vi "Performance Test.vi"() -> ()   [LabVIEW 2021]
uses:
  <vilib>/Platform/TimedLoop/XDataNode/wakeup.ctl
  <vilib>/Platform/TimedLoop/XDataNode/XDNodeRunTimeDep.lvlib
  <vilib>/Platform/TimedLoop/XDataNode/nitl_modes.ctl
  <vilib>/Platform/TimedLoop/XDataNode/timing_clust.ctl
  <vilib>/Platform/TimedLoop/XDataNode/XDataNode.xnode
  CIFChannels/Typedef/Direction.ctl
  CIFChannels/CIFChannels.lvclass
  ChannelCommon/typedef/FIFO Config.ctl
  ChannelCommon/ChannelCommon.lvlib
  ChannelRegistrar/typedef/Datatype CAN.ctl
  ChannelRegistrar/ChannelRegistrar.lvlib
  CIF_NIChn_FifoCAN.lvclass
  D:/dev/CIF-LVCore/src/Channels/CIF_NIChn/NIChn/CIF_NIChn.lvclass
  D:/dev/CIF-LVCore/src/Channels/CIFChannels/CIFChannels.lvclass
  D:/dev/CIF-LVCore/src/Channels/CIF_NIChn/FIFO_CAN/CIF_NIChn_FifoCAN.lvclass
panel:
  out "avg CAN_TO":dbl
  out "max CAN_TO":dbl
  out "timed out? 3":bool
  out "avg CAN_Direct":dbl
  out "max CAN_Direct":dbl
  out "timed out? 2":bool
  out "timed out?":bool
  out "avg CAN channel":dbl
  out "max CAN channel":dbl
  out "pass":bool
  out "error out":errorcluster
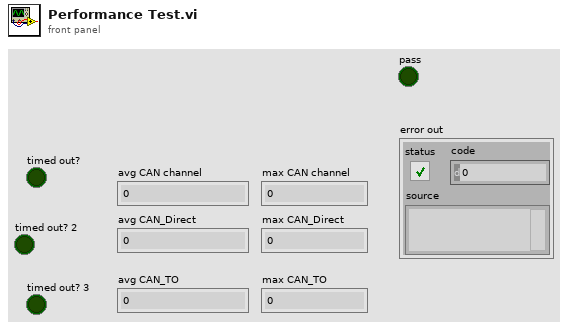
[diagram p1: front panel]
types:
  T1 = typedef "ChannelCommon.lvlib/FIFO Config.ctl" = cluster{"Depth":u64, "Flags":u64}
  T2 = typedef "CIFChannels.lvclass/Direction.ctl" = enum16{"Publisher", "Subscriber"}
  T3 = typedef "ChannelRegistrar.lvlib/Datatype CAN.ctl" = cluster{"payload":u8[], "identifier":u32, "Tags":u8, "Timestamp":u64}
  T4 = typedef "XDNodeRunTimeDep.lvlib/timing_clust.ctl" = cluster{"Expected End [f-1]":u64, "Actual End [f-1]":u64, "Finished Late? [f-1]":bool, "Expected End [i-1]":u64, "Actual End [i-1]":u64, "Finished Late? [i-1]":bool, "Expected Start [i]":u64, "Actual Start [i]":u64, "Expected Start [f]":u64, "Actual Start [f]":u64, "Source Name":string, "Structure Name":string, "Period":i64, "Deadline":i64, "Offset":i64, "Start":i64, "Priority":i32, "Timeout":i32, "Mode":T5, "Wakeup Reason":T6, "Error":errorcluster, "Source Type":string, "Secondary Source Type":string, "Global End Time":u64, "Global Start Time":u64, "Frame Duration":u64, "Iteration Duration":u64, "Assigned CPU":i32, "I/O Scan Engine Mode":u32}
  T5 = typedef "XDNodeRunTimeDep.lvlib/nitl_modes.ctl" = enum32{"No Change", "Process missed periods, maintain original phase", "Discard missed periods, maintain original phase", "Process missed periods, ignore original phase", "Discard missed periods, ignore original phase"}
  T6 = typedef "XDNodeRunTimeDep.lvlib/wakeup.ctl" = enum32{"Normal", "Aborted", "Asynchronous wakeup", "Timing source error", "Timed loop error", "Timeout"}
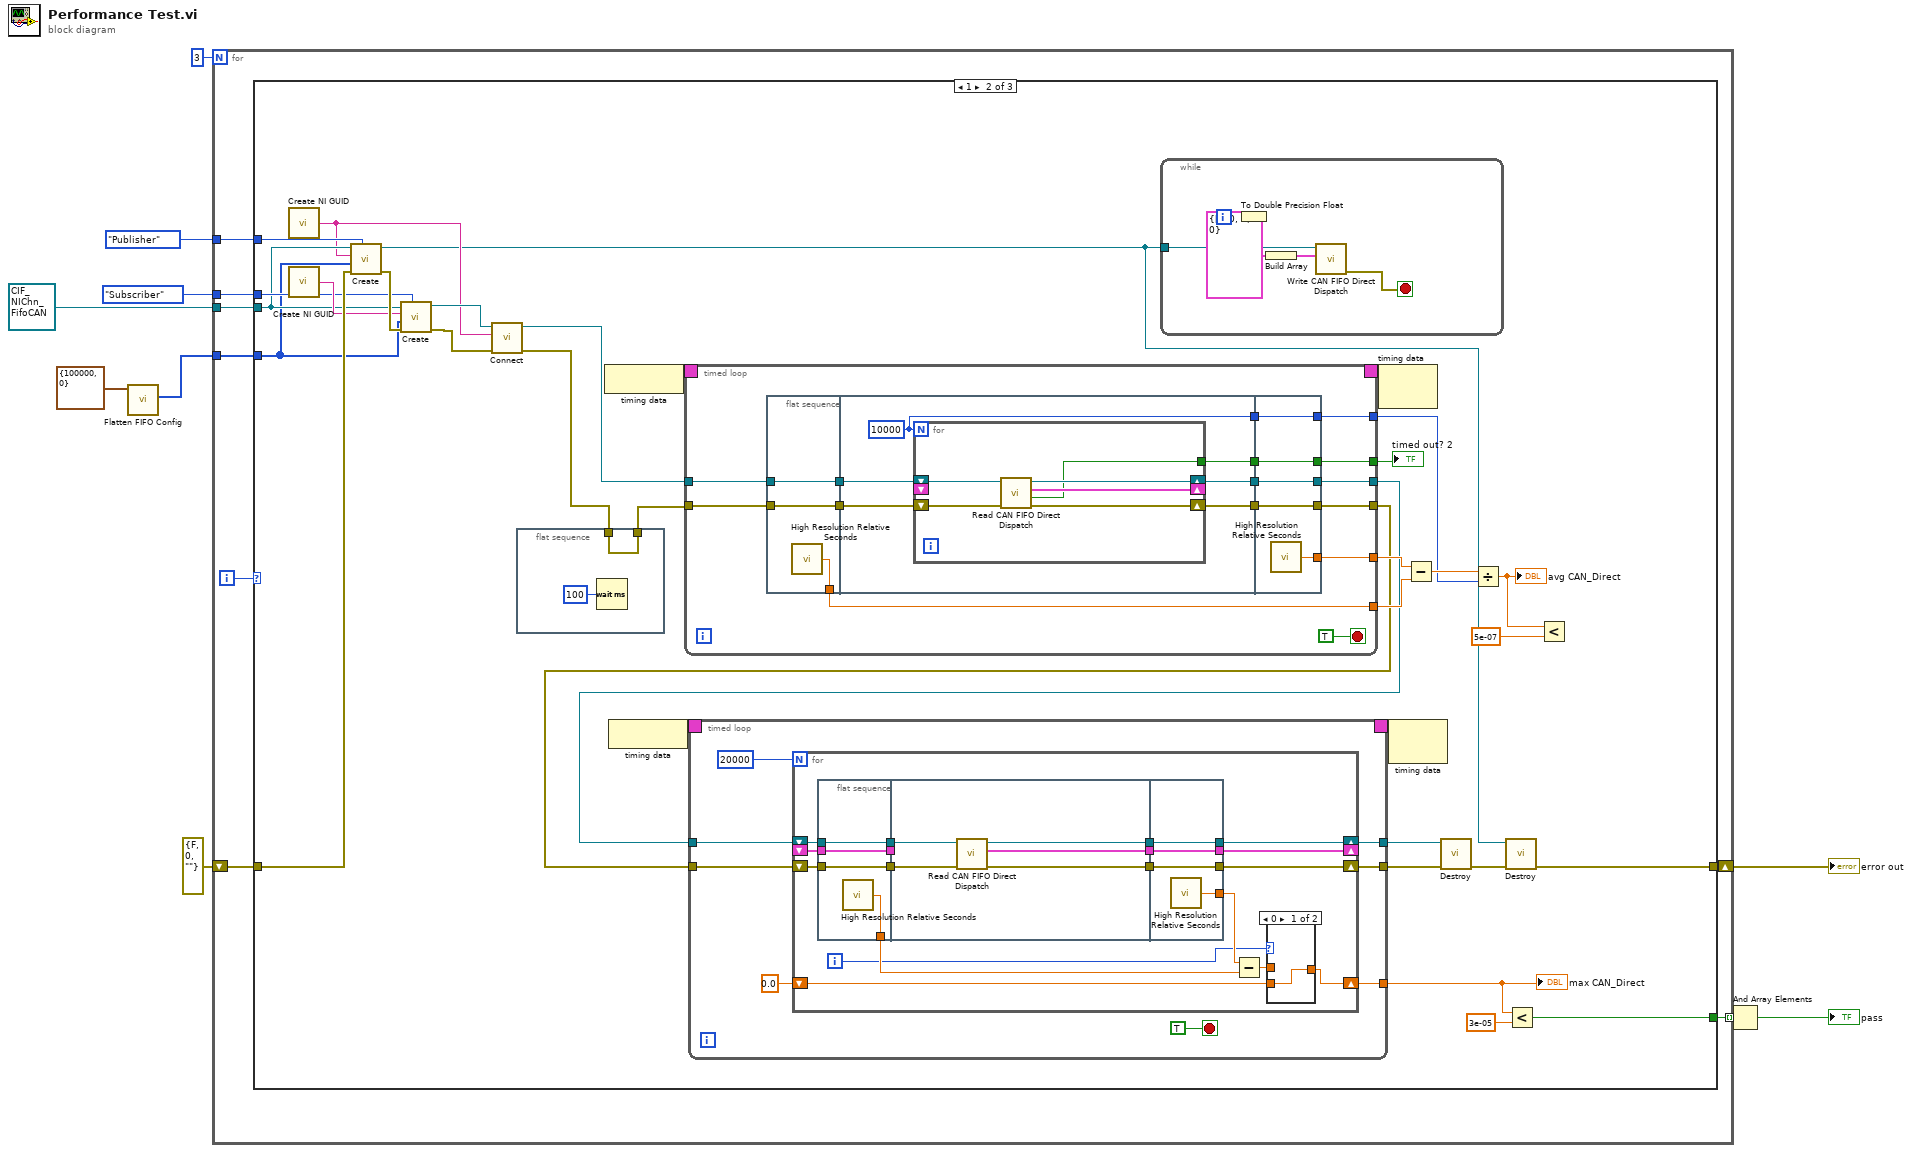
[diagram p0: block diagram]
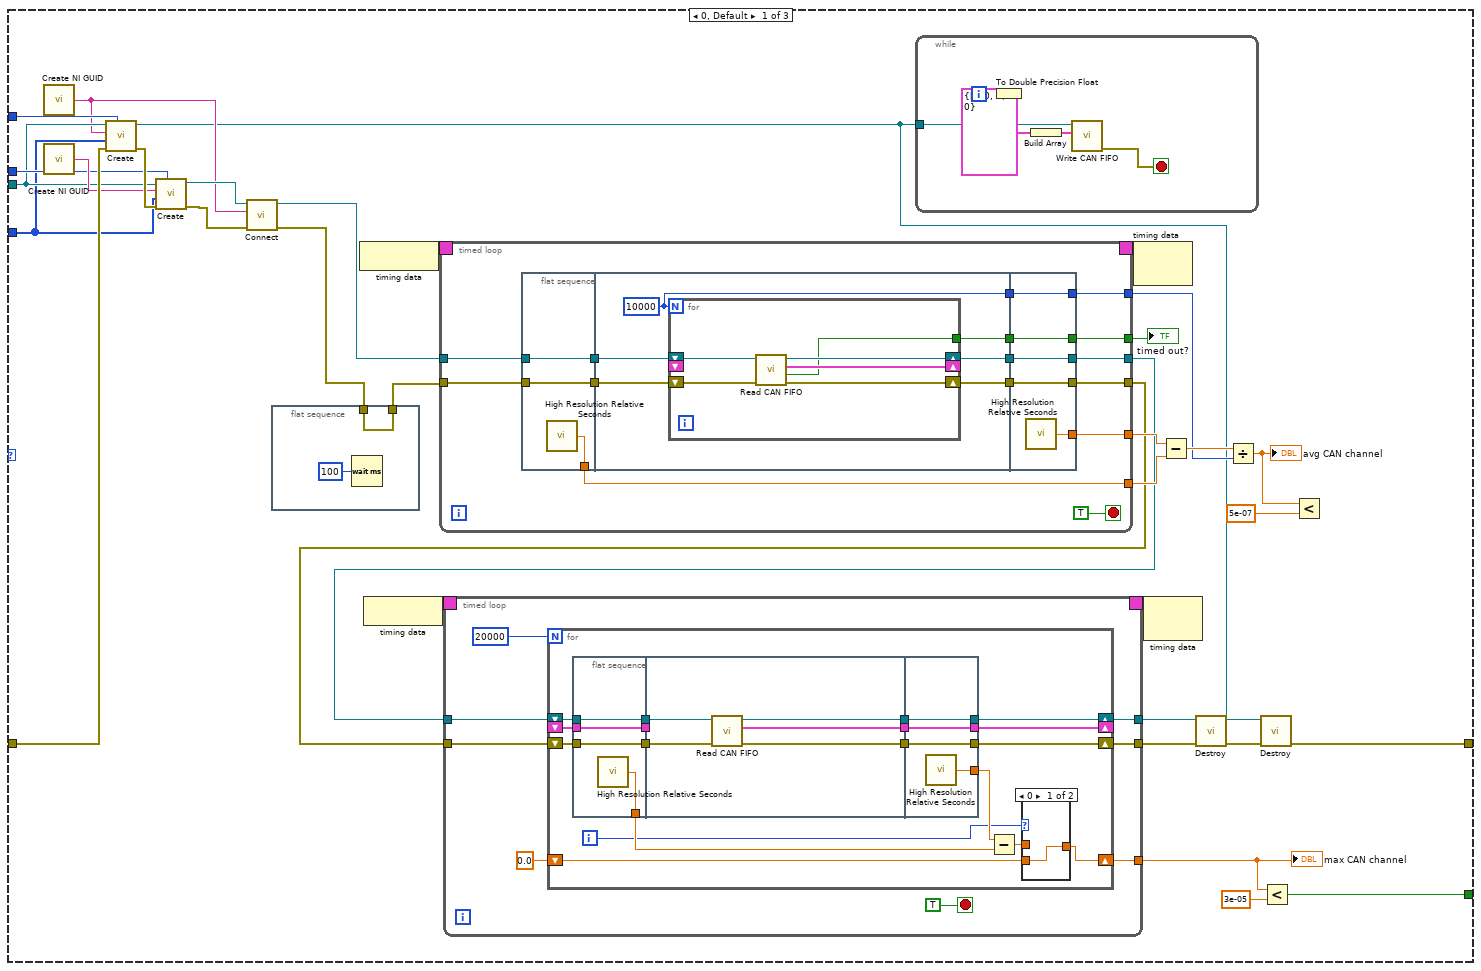
[diagram p2: hidden frame]
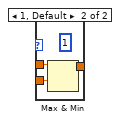
[diagram p3: hidden frame]
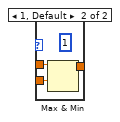
[diagram p4: hidden frame]
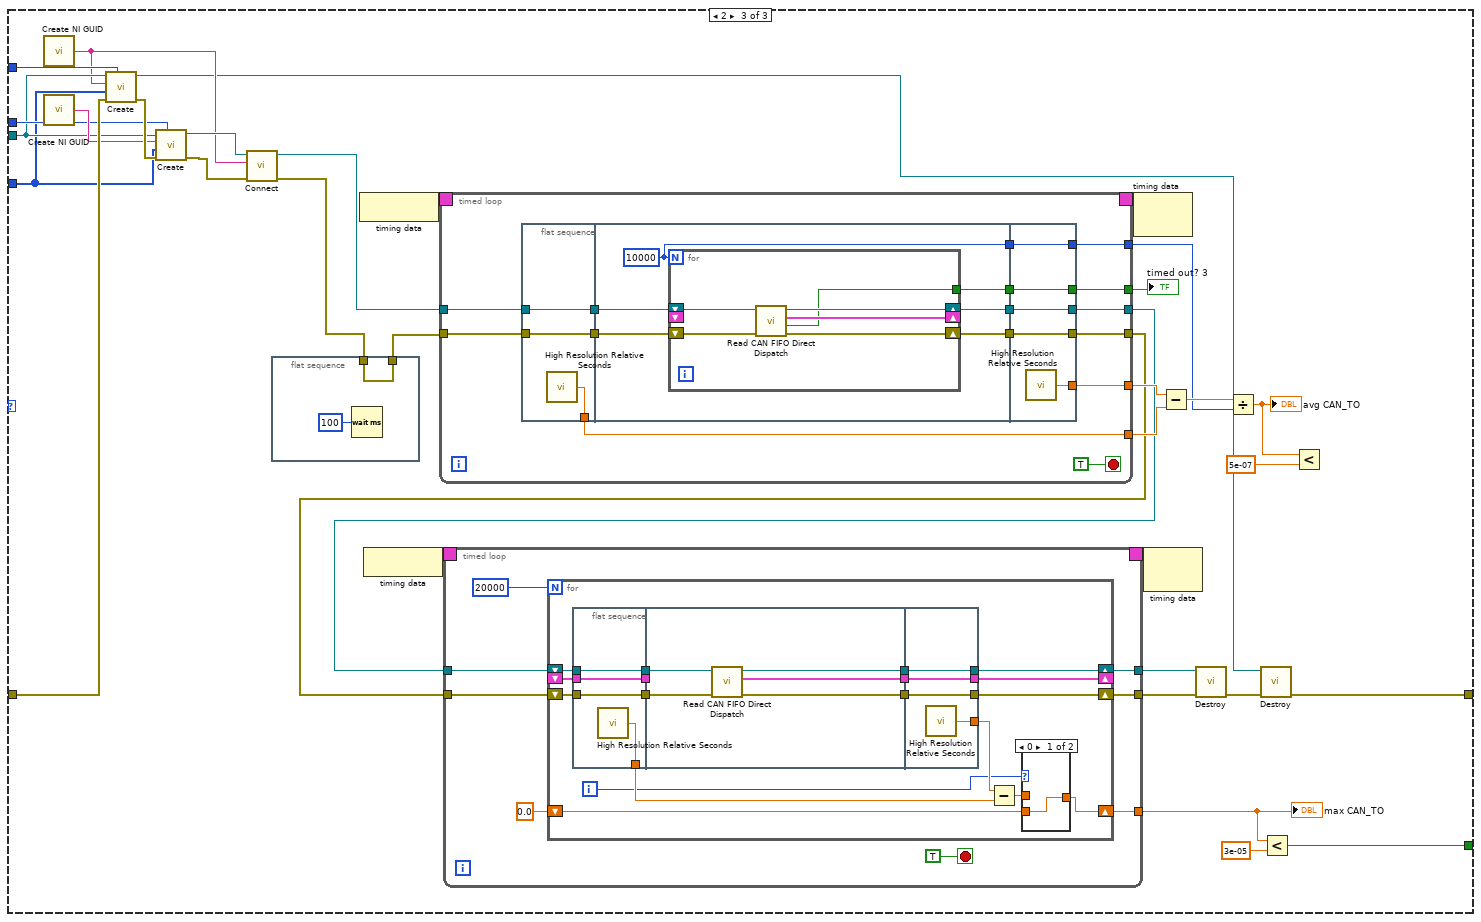
[diagram p5: hidden frame]
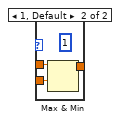
[diagram p6: hidden frame]
diagram:
  n1 = call "Flatten FIFO Config.vi"("FIFO Config in"=T1 {"Depth"=100000, "Flags"=0}) -> ("Flattened Data out"=w2:u8[])  [unwired: 8 in, 2 out]
  n2 = for {
    N: 3 -> [_]
    tunnel: [w18] -> w8 mode=indexing
    shift-right: [w17] -> w10
    shift-left: errorcluster {"status"=FALSE, "code"=0, "source"=""} ("error out") -> [w15]
    tunnel: Direction."Publisher" ("Direction") -> [w14]
    tunnel: Direction."Subscriber" ("Direction") -> [w13]
    tunnel: refnum<class "CIF_NIChn_FifoCAN.lvclass"> refnum ("CIF_NIChn_FifoCAN.lvclass") -> [w12]
    tunnel: w2 -> [w11]
    i -> [w16]
    n3 = case shown="1" w16 {
      tunnel: [w38 w165 w292] -> w18
      tunnel: [w22 w149 w276] -> w17
      tunnel: w15 -> [w36 w163 w290]
      tunnel: w14 -> [w34 w161 w288]
      tunnel: w13 -> [w33 w160 w287]
      tunnel: w12 -> [w32 w159 w286]
      tunnel: w11 -> [w28 w155 w282]
      frame 0, Default {
        n4 = call <vilib>:"Create NI GUID.vi"() -> ("NI GUID"=w30:string)
        n5 = call <vilib>:"Create NI GUID.vi"() -> ("NI GUID"=w35:string)
        n6 = call-dynamic "Create.vi"("Direction"=w34, "error in (no error)"=w36, "Custom Config Data"=w28, "Name"=w30, "CIFTag in"=w32) -> ("error out"=w37:errorcluster, "CIFTag out"=w23:refnum<class "CIF_NIChn_FifoCAN.lvclass">)  [unwired: 5 in]
        n7 = call-dynamic "Create.vi"("Direction"=w33, "error in (no error)"=w37, "Custom Config Data"=w28, "Name"=w35, "CIFTag in"=w32) -> ("error out"=w29:errorcluster, "CIFTag out"=w31:refnum<class "CIF_NIChn_FifoCAN.lvclass">)  [unwired: 5 in]
        n8 = call-dynamic "Connect.vi"("error in (no error)"=w29, "Connection Name"=w30, "CIFTag in"=w31) -> ("error out"=w21:errorcluster, "CIFTag out"=w27:refnum<class "CIF_NIChn_FifoCAN.lvclass">)  [unwired: 7 in]
        n9 = flat-sequence {
          tunnel: w21 -> [w54]
          tunnel: [w54] -> w20
          frame #0 {
            n10 = Wait (ms)(milliseconds to wait=u32 100) -> ()  [unwired: 1 out]
          }
        }
        n11 = node-c288() -> (w52:T4)
        n12 = node-c288() -> (w50:T4)
        n13 = timed-loop {
          timing: w52 -> [_]
          timing-out: [_] -> w51
          tunnel: w27 -> [w121]
          tunnel: w20 -> [w120]
          tunnel: [w116] -> w44
          tunnel: [w114] -> w43
          tunnel: [w112] -> w48
          tunnel: [w111] -> w47
          tunnel: [w110] -> w45
          tunnel: [w108] -> w19
          stop <- TRUE stop-if-true
          n14 = flat-sequence {
            tunnel: w120 -> [w123]
            tunnel: w121 -> [w124]
            tunnel: [w124] -> w118
            tunnel: [w123] -> w117
            tunnel: [w122] -> w111
            tunnel: w118 -> [w130]
            tunnel: w117 -> [w129]
            tunnel: [w128] -> w115
            tunnel: [w127] -> w113
            tunnel: [w126] -> w109
            tunnel: [w125] -> w107
            tunnel: [w141] -> w116
            tunnel: w115 -> [w141]
            tunnel: [w140] -> w114
            tunnel: w113 -> [w140]
            tunnel: [w139] -> w112
            tunnel: [w138] -> w110
            tunnel: w109 -> [w138]
            tunnel: [w137] -> w108
            tunnel: w107 -> [w137]
            frame #0 {
              n15 = call <vilib>:"High Resolution Relative Seconds.vi"() -> ("relative seconds"=w122:dbl)
            }
            frame #1 {
              w126 = 10000
              n16 = for {
                N: w126 -> [_]
                shift-right: [w135] -> w128
                shift-left: w130 -> [w136]
                shift-right: [w133] -> w127
                shift-left: w129 -> [w134]
                shift-right: [w132] -> _
                shift-left: _ -> [_]
                tunnel: [w131] -> w125
                n17 = call-dynamic "Read CAN FIFO.vi"("error in (no error)"=w134, "CIFTag in"=w136) -> ("error out"=w133:errorcluster, "timed out?"=w131:bool, "Data"=w132:T3[], "CIFTag out"=w135:refnum<class "CIF_NIChn_FifoCAN.lvclass">)  [unwired: 5 in, 1 out]
              }
            }
            frame #2 {
              n18 = call <vilib>:"High Resolution Relative Seconds.vi"() -> ("relative seconds"=w139:dbl)
            }
          }
        }
        "timed out?" <- w19
        n19 = timed-loop {
          timing: w50 -> [_]
          timing-out: [_] -> w49
          tunnel: w44 -> [w67]
          tunnel: w43 -> [w66]
          tunnel: [w64] -> w26
          tunnel: [w63] -> w25
          tunnel: [w60] -> w40
          stop <- TRUE stop-if-true
          n20 = for {
            N: 20000 -> [_]
            shift-right: [w79] -> w64
            shift-left: w67 -> [w81]
            shift-right: [w78] -> w63
            shift-left: w66 -> [w80]
            shift-right: [w72] -> w60
            shift-left: 0.0 -> [w73]
            shift-right: [w71] -> _
            shift-left: _ -> [w77]
            i -> [w69]
            n21 = flat-sequence {
              tunnel: w80 -> [w92]
              tunnel: w81 -> [w93]
              tunnel: [w93] -> w85
              tunnel: [w92] -> w84
              tunnel: [w91] -> w75
              tunnel: w77 -> [w90]
              tunnel: [w90] -> w83
              tunnel: w85 -> [w98]
              tunnel: w84 -> [w96]
              tunnel: [w97] -> w82
              tunnel: w83 -> [_]
              tunnel: [w94] -> w70
              tunnel: [w95] -> w68
              tunnel: [w102] -> w79
              tunnel: w82 -> [w102]
              tunnel: [w101] -> w78
              tunnel: [w100] -> w76
              tunnel: [w99] -> w71
              tunnel: w70 -> [w99]
              tunnel: w68 -> [w101]
              frame #0 {
                n22 = call <vilib>:"High Resolution Relative Seconds.vi"() -> ("relative seconds"=w91:dbl)
              }
              frame #1 {
                n23 = call-dynamic "Read CAN FIFO.vi"("error in (no error)"=w96, "CIFTag in"=w98) -> ("error out"=w95:errorcluster, "Data"=w94:T3[], "CIFTag out"=w97:refnum<class "CIF_NIChn_FifoCAN.lvclass">)  [unwired: 5 in, 2 out]
              }
              frame #2 {
                n24 = call <vilib>:"High Resolution Relative Seconds.vi"() -> ("relative seconds"=w100:dbl)
              }
            }
            n25 = Subtract(x=w76, y=w75) -> (x-y=w74:dbl)
            n26 = case shown="0" w69 {
              tunnel: w74 -> [_ w89]
              tunnel: w73 -> [w86 w88]
              tunnel: [w86 w87] -> w72
              frame 0 {
              }
              frame 1, Default {
                (unwired) u32 1 ("milliseconds to wait")
                n27 = Max & Min(x=w89, y=w88) -> (max(x,y)=w87:dbl)  [unwired: 1 out]
              }
            }
          }
        }
        "max CAN channel" <- w40
        n28 = while {
          tunnel: w23 -> [w58]
          i -> [w59]
          stop <- w56 stop-if-true
          n29 = To Double Precision Float(number=w59) -> ()  [unwired: 1 out]
          n30 = Build Array(T3 {"payload"=[], "identifier"=0, "Tags"=0, "Timestamp"=0} ("Data")) -> (w55:T3[])
          n31 = call-dynamic "Write CAN FIFO.vi"("Data"=w55, "CIFTag in"=w58) -> ("error out"=w56:errorcluster)  [unwired: 7 in, 2 out]
        }
        n32 = node-c288(w51) -> ()  [unwired: 1 out]
        n33 = node-c288(w49) -> ()  [unwired: 1 out]
        n34 = Subtract(x=w48, y=w47) -> (x-y=w46:dbl)
        n35 = call-dynamic "Destroy.vi"("error in (no error)"=w25, "CIFTag in"=w26) -> ("error out"=w24:errorcluster)  [unwired: 8 in, 1 out]
        n36 = Divide(x=w46, y=w45) -> (x/y=w42:dbl)
        "avg CAN channel" <- w42
        n37 = call-dynamic "Destroy.vi"("error in (no error)"=w24, "CIFTag in"=w23) -> ("error out"=w22:errorcluster)  [unwired: 8 in, 1 out]
        n38 = Less?(x=w40, y=3e-05) -> (x < y?=w38:bool)
        n39 = Less?(x=w42, y=5e-07) -> ()  [unwired: 1 out]
      }
      frame 1 {
        n40 = call <vilib>:"Create NI GUID.vi"() -> ("NI GUID"=w157:string)
        n41 = call <vilib>:"Create NI GUID.vi"() -> ("NI GUID"=w162:string)
        n42 = call-dynamic "Create.vi"("Direction"=w161, "error in (no error)"=w163, "Custom Config Data"=w155, "Name"=w157, "CIFTag in"=w159) -> ("error out"=w164:errorcluster, "CIFTag out"=w150:refnum<class "CIF_NIChn_FifoCAN.lvclass">)  [unwired: 5 in]
        n43 = call-dynamic "Create.vi"("Direction"=w160, "error in (no error)"=w164, "Custom Config Data"=w155, "Name"=w162, "CIFTag in"=w159) -> ("error out"=w156:errorcluster, "CIFTag out"=w158:refnum<class "CIF_NIChn_FifoCAN.lvclass">)  [unwired: 5 in]
        n44 = call-dynamic "Connect.vi"("error in (no error)"=w156, "Connection Name"=w157, "CIFTag in"=w158) -> ("error out"=w148:errorcluster, "CIFTag out"=w154:refnum<class "CIF_NIChn_FifoCAN.lvclass">)  [unwired: 7 in]
        n45 = flat-sequence {
          tunnel: w148 -> [w181]
          tunnel: [w181] -> w147
          frame #0 {
            n46 = Wait (ms)(milliseconds to wait=u32 100) -> ()  [unwired: 1 out]
          }
        }
        n47 = node-c288() -> (w179:T4)
        n48 = node-c288() -> (w177:T4)
        n49 = timed-loop {
          timing: w179 -> [_]
          timing-out: [_] -> w178
          tunnel: w154 -> [w248]
          tunnel: w147 -> [w247]
          tunnel: [w243] -> w171
          tunnel: [w241] -> w170
          tunnel: [w239] -> w175
          tunnel: [w238] -> w174
          tunnel: [w237] -> w172
          tunnel: [w235] -> w146
          stop <- TRUE stop-if-true
          n50 = flat-sequence {
            tunnel: w247 -> [w250]
            tunnel: w248 -> [w251]
            tunnel: [w251] -> w245
            tunnel: [w250] -> w244
            tunnel: [w249] -> w238
            tunnel: w245 -> [w257]
            tunnel: w244 -> [w256]
            tunnel: [w255] -> w242
            tunnel: [w254] -> w240
            tunnel: [w253] -> w236
            tunnel: [w252] -> w234
            tunnel: [w268] -> w243
            tunnel: w242 -> [w268]
            tunnel: [w267] -> w241
            tunnel: w240 -> [w267]
            tunnel: [w266] -> w239
            tunnel: [w265] -> w237
            tunnel: w236 -> [w265]
            tunnel: [w264] -> w235
            tunnel: w234 -> [w264]
            frame #0 {
              n51 = call <vilib>:"High Resolution Relative Seconds.vi"() -> ("relative seconds"=w249:dbl)
            }
            frame #1 {
              w253 = 10000
              n52 = for {
                N: w253 -> [_]
                shift-right: [w262] -> w255
                shift-left: w257 -> [w263]
                shift-right: [w260] -> w254
                shift-left: w256 -> [w261]
                shift-right: [w259] -> _
                shift-left: _ -> [_]
                tunnel: [w258] -> w252
                n53 = call "Read CAN FIFO Direct Dispatch.vi"("error in (no error)"=w261, "CIFTag in"=w263) -> ("error out"=w260:errorcluster, "timed out?"=w258:bool, "Data"=w259:T3[], "CIFTag out"=w262:refnum<class "CIF_NIChn_FifoCAN.lvclass">)  [unwired: 5 in, 1 out]
              }
            }
            frame #2 {
              n54 = call <vilib>:"High Resolution Relative Seconds.vi"() -> ("relative seconds"=w266:dbl)
            }
          }
        }
        "timed out? 2" <- w146
        n55 = timed-loop {
          timing: w177 -> [_]
          timing-out: [_] -> w176
          tunnel: w171 -> [w194]
          tunnel: w170 -> [w193]
          tunnel: [w191] -> w153
          tunnel: [w190] -> w152
          tunnel: [w187] -> w167
          stop <- TRUE stop-if-true
          n56 = for {
            N: 20000 -> [_]
            shift-right: [w206] -> w191
            shift-left: w194 -> [w208]
            shift-right: [w205] -> w190
            shift-left: w193 -> [w207]
            shift-right: [w199] -> w187
            shift-left: 0.0 -> [w200]
            shift-right: [w198] -> _
            shift-left: _ -> [w204]
            i -> [w196]
            n57 = flat-sequence {
              tunnel: w207 -> [w219]
              tunnel: w208 -> [w220]
              tunnel: [w220] -> w212
              tunnel: [w219] -> w211
              tunnel: [w218] -> w202
              tunnel: w204 -> [w217]
              tunnel: [w217] -> w210
              tunnel: w212 -> [w225]
              tunnel: w211 -> [w223]
              tunnel: [w224] -> w209
              tunnel: w210 -> [_]
              tunnel: [w221] -> w197
              tunnel: [w222] -> w195
              tunnel: [w229] -> w206
              tunnel: w209 -> [w229]
              tunnel: [w228] -> w205
              tunnel: [w227] -> w203
              tunnel: [w226] -> w198
              tunnel: w197 -> [w226]
              tunnel: w195 -> [w228]
              frame #0 {
                n58 = call <vilib>:"High Resolution Relative Seconds.vi"() -> ("relative seconds"=w218:dbl)
              }
              frame #1 {
                n59 = call "Read CAN FIFO Direct Dispatch.vi"("error in (no error)"=w223, "CIFTag in"=w225) -> ("error out"=w222:errorcluster, "Data"=w221:T3[], "CIFTag out"=w224:refnum<class "CIF_NIChn_FifoCAN.lvclass">)  [unwired: 5 in, 2 out]
              }
              frame #2 {
                n60 = call <vilib>:"High Resolution Relative Seconds.vi"() -> ("relative seconds"=w227:dbl)
              }
            }
            n61 = Subtract(x=w203, y=w202) -> (x-y=w201:dbl)
            n62 = case shown="0" w196 {
              tunnel: w201 -> [_ w216]
              tunnel: w200 -> [w213 w215]
              tunnel: [w213 w214] -> w199
              frame 0 {
              }
              frame 1, Default {
                (unwired) u32 1 ("milliseconds to wait")
                n63 = Max & Min(x=w216, y=w215) -> (max(x,y)=w214:dbl)  [unwired: 1 out]
              }
            }
          }
        }
        "max CAN_Direct" <- w167
        n64 = while {
          tunnel: w150 -> [w185]
          i -> [w186]
          stop <- w183 stop-if-true
          n65 = To Double Precision Float(number=w186) -> ()  [unwired: 1 out]
          n66 = Build Array(T3 {"payload"=[], "identifier"=0, "Tags"=0, "Timestamp"=0} ("Data")) -> (w182:T3[])
          n67 = call "Write CAN FIFO Direct Dispatch.vi"("Data"=w182, "CIFTag in"=w185) -> ("error out"=w183:errorcluster)  [unwired: 7 in, 2 out]
        }
        n68 = node-c288(w178) -> ()  [unwired: 1 out]
        n69 = node-c288(w176) -> ()  [unwired: 1 out]
        n70 = Subtract(x=w175, y=w174) -> (x-y=w173:dbl)
        n71 = call-dynamic "Destroy.vi"("error in (no error)"=w152, "CIFTag in"=w153) -> ("error out"=w151:errorcluster)  [unwired: 8 in, 1 out]
        n72 = Divide(x=w173, y=w172) -> (x/y=w169:dbl)
        "avg CAN_Direct" <- w169
        n73 = call-dynamic "Destroy.vi"("error in (no error)"=w151, "CIFTag in"=w150) -> ("error out"=w149:errorcluster)  [unwired: 8 in, 1 out]
        n74 = Less?(x=w167, y=3e-05) -> (x < y?=w165:bool)
        n75 = Less?(x=w169, y=5e-07) -> ()  [unwired: 1 out]
      }
      frame 2 {
        n76 = call <vilib>:"Create NI GUID.vi"() -> ("NI GUID"=w284:string)
        n77 = call <vilib>:"Create NI GUID.vi"() -> ("NI GUID"=w289:string)
        n78 = call-dynamic "Create.vi"("Direction"=w288, "error in (no error)"=w290, "Custom Config Data"=w282, "Name"=w284, "CIFTag in"=w286) -> ("error out"=w291:errorcluster, "CIFTag out"=w277:refnum<class "CIF_NIChn_FifoCAN.lvclass">)  [unwired: 5 in]
        n79 = call-dynamic "Create.vi"("Direction"=w287, "error in (no error)"=w291, "Custom Config Data"=w282, "Name"=w289, "CIFTag in"=w286) -> ("error out"=w283:errorcluster, "CIFTag out"=w285:refnum<class "CIF_NIChn_FifoCAN.lvclass">)  [unwired: 5 in]
        n80 = call-dynamic "Connect.vi"("error in (no error)"=w283, "Connection Name"=w284, "CIFTag in"=w285) -> ("error out"=w275:errorcluster, "CIFTag out"=w281:refnum<class "CIF_NIChn_FifoCAN.lvclass">)  [unwired: 7 in]
        n81 = flat-sequence {
          tunnel: w275 -> [w308]
          tunnel: [w308] -> w274
          frame #0 {
            n82 = Wait (ms)(milliseconds to wait=u32 100) -> ()  [unwired: 1 out]
          }
        }
        n83 = node-c288() -> (w306:T4)
        n84 = node-c288() -> (w304:T4)
        n85 = timed-loop {
          timing: w306 -> [_]
          timing-out: [_] -> w305
          tunnel: w281 -> [w370]
          tunnel: w274 -> [w369]
          tunnel: [w365] -> w298
          tunnel: [w363] -> w297
          tunnel: [w361] -> w302
          tunnel: [w360] -> w301
          tunnel: [w359] -> w299
          tunnel: [w357] -> w273
          stop <- TRUE stop-if-true
          n86 = flat-sequence {
            tunnel: w369 -> [w372]
            tunnel: w370 -> [w373]
            tunnel: [w373] -> w367
            tunnel: [w372] -> w366
            tunnel: [w371] -> w360
            tunnel: w367 -> [w379]
            tunnel: w366 -> [w378]
            tunnel: [w377] -> w364
            tunnel: [w376] -> w362
            tunnel: [w375] -> w358
            tunnel: [w374] -> w356
            tunnel: [w390] -> w365
            tunnel: w364 -> [w390]
            tunnel: [w389] -> w363
            tunnel: w362 -> [w389]
            tunnel: [w388] -> w361
            tunnel: [w387] -> w359
            tunnel: w358 -> [w387]
            tunnel: [w386] -> w357
            tunnel: w356 -> [w386]
            frame #0 {
              n87 = call <vilib>:"High Resolution Relative Seconds.vi"() -> ("relative seconds"=w371:dbl)
            }
            frame #1 {
              w375 = 10000
              n88 = for {
                N: w375 -> [_]
                shift-right: [w384] -> w377
                shift-left: w379 -> [w385]
                shift-right: [w382] -> w376
                shift-left: w378 -> [w383]
                shift-right: [w381] -> _
                shift-left: _ -> [_]
                tunnel: [w380] -> w374
                n89 = call "Read CAN FIFO Direct Dispatch.vi"("error in (no error)"=w383, "CIFTag in"=w385) -> ("error out"=w382:errorcluster, "timed out?"=w380:bool, "Data"=w381:T3[], "CIFTag out"=w384:refnum<class "CIF_NIChn_FifoCAN.lvclass">)  [unwired: 5 in, 1 out]
              }
            }
            frame #2 {
              n90 = call <vilib>:"High Resolution Relative Seconds.vi"() -> ("relative seconds"=w388:dbl)
            }
          }
        }
        "timed out? 3" <- w273
        n91 = timed-loop {
          timing: w304 -> [_]
          timing-out: [_] -> w303
          tunnel: w298 -> [w316]
          tunnel: w297 -> [w315]
          tunnel: [w313] -> w280
          tunnel: [w312] -> w279
          tunnel: [w309] -> w294
          stop <- TRUE stop-if-true
          n92 = for {
            N: 20000 -> [_]
            shift-right: [w328] -> w313
            shift-left: w316 -> [w330]
            shift-right: [w327] -> w312
            shift-left: w315 -> [w329]
            shift-right: [w321] -> w309
            shift-left: 0.0 -> [w322]
            shift-right: [w320] -> _
            shift-left: _ -> [w326]
            i -> [w318]
            n93 = flat-sequence {
              tunnel: w329 -> [w341]
              tunnel: w330 -> [w342]
              tunnel: [w342] -> w334
              tunnel: [w341] -> w333
              tunnel: [w340] -> w324
              tunnel: w326 -> [w339]
              tunnel: [w339] -> w332
              tunnel: w334 -> [w347]
              tunnel: w333 -> [w345]
              tunnel: [w346] -> w331
              tunnel: w332 -> [_]
              tunnel: [w343] -> w319
              tunnel: [w344] -> w317
              tunnel: [w351] -> w328
              tunnel: w331 -> [w351]
              tunnel: [w350] -> w327
              tunnel: [w349] -> w325
              tunnel: [w348] -> w320
              tunnel: w319 -> [w348]
              tunnel: w317 -> [w350]
              frame #0 {
                n94 = call <vilib>:"High Resolution Relative Seconds.vi"() -> ("relative seconds"=w340:dbl)
              }
              frame #1 {
                n95 = call "Read CAN FIFO Direct Dispatch.vi"("error in (no error)"=w345, "CIFTag in"=w347) -> ("error out"=w344:errorcluster, "Data"=w343:T3[], "CIFTag out"=w346:refnum<class "CIF_NIChn_FifoCAN.lvclass">)  [unwired: 5 in, 2 out]
              }
              frame #2 {
                n96 = call <vilib>:"High Resolution Relative Seconds.vi"() -> ("relative seconds"=w349:dbl)
              }
            }
            n97 = Subtract(x=w325, y=w324) -> (x-y=w323:dbl)
            n98 = case shown="0" w318 {
              tunnel: w323 -> [_ w338]
              tunnel: w322 -> [w335 w337]
              tunnel: [w335 w336] -> w321
              frame 0 {
              }
              frame 1, Default {
                (unwired) u32 1 ("milliseconds to wait")
                n99 = Max & Min(x=w338, y=w337) -> (max(x,y)=w336:dbl)  [unwired: 1 out]
              }
            }
          }
        }
        "max CAN_TO" <- w294
        n100 = node-c288(w305) -> ()  [unwired: 1 out]
        n101 = node-c288(w303) -> ()  [unwired: 1 out]
        n102 = Subtract(x=w302, y=w301) -> (x-y=w300:dbl)
        n103 = call-dynamic "Destroy.vi"("error in (no error)"=w279, "CIFTag in"=w280) -> ("error out"=w278:errorcluster)  [unwired: 8 in, 1 out]
        n104 = Divide(x=w300, y=w299) -> (x/y=w296:dbl)
        "avg CAN_TO" <- w296
        n105 = call-dynamic "Destroy.vi"("error in (no error)"=w278, "CIFTag in"=w277) -> ("error out"=w276:errorcluster)  [unwired: 8 in, 1 out]
        n106 = Less?(x=w294, y=3e-05) -> (x < y?=w292:bool)
        n107 = Less?(x=w296, y=5e-07) -> ()  [unwired: 1 out]
      }
    }
  }
  "error out" <- w10
  n108 = And Array Elements(Boolean array=w8) -> (logical AND=→"pass":bool)
